vi "MoveNext.vi"(8 "error in (no error)":errorcluster caption="错误输入（无错误）", 11 "Enumerator 输入":refnum<class "Enumerator.lvclass"> caption="DNL_LabVIEW Object in") -> (0 "error out":errorcluster caption="错误输出", 2 "MoveNext":bool, 3 "Enumerator 输出":refnum<class "Enumerator.lvclass"> caption="DNL_LabVIEW Object out")   [LabVIEW 2012, in "Enumerator.lvclass"]
uses:
  Enumerator.lvclass
  Enumerator.lvclass/Enumerator.ctl
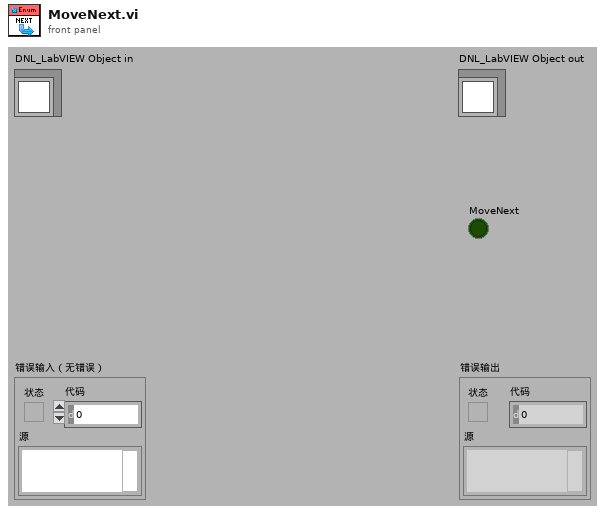
[diagram p1: front panel]
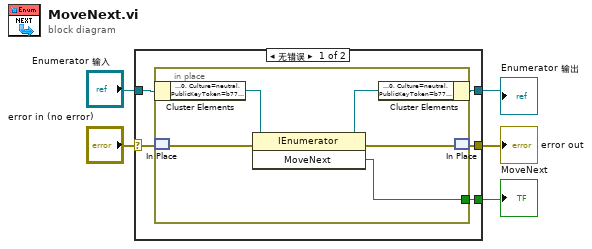
[diagram p0: block diagram]
diagram:
  n1 = case shown="无错误" "error in (no error)" {
    selector: "error in (no error)" -> [w9 w17]
    tunnel: [w6 w17] -> w4
    tunnel: [w7 w16] -> w2
    tunnel: "Enumerator 输入" -> [w10 w16]
    tunnel: [w8 _] -> w1
    frame No Error {
      n2 = in-place {
        in-place-border: [w13] -> w8
        n3 = in-place-cluster #1(w10) -> ("Enumerator"=w15:refnum<k24>)
        n4 = in-place-match #2(w9) -> (w12:errorcluster)
        n5 = invoke class="IEnumerator" method="MoveNext"(reference=w15, error in=w12) -> (reference out=w14:refnum<k24>, error out=w11:errorcluster, "MoveNext"=w13:bool)  [unwired: 1 in]
        n6 = in-place-cluster #1("Enumerator"=w14) -> (w7:refnum<class "Enumerator.lvclass">)
        n7 = in-place-match #2(w11) -> (w6:errorcluster)
      }
    }
    frame Error {
    }
  }
  "error out" <- w4
  "Enumerator 输出" <- w2
  "MoveNext" <- w1
